vi "enable-ui-element.vi"(2 "Enable UI Element":bool) -> (7 "UI Element State":T1(ring))   [LabVIEW 2024]
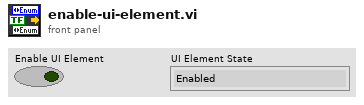
[diagram p1: front panel]
types:
  T1 = enum8{"Enabled", "Disabled", "Disabled and Grayed Out"}
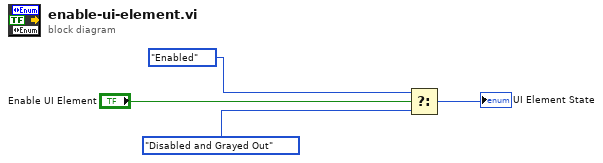
[diagram p0: block diagram]
diagram:
  n1 = Select(t=T1."Enabled" ("Disabled"), s="Enable UI Element", f=T1."Disabled and Grayed Out" ("Disabled")) -> (s? t:f=→"UI Element State":T1)
